vi "test_pattern_recognition.vi"() -> ()   [LabVIEW 2015]
panel:
  out "Matches (pixel) 2":T1(array[cluster])
  in  "Imaginea":path
  in  "Path to template":path
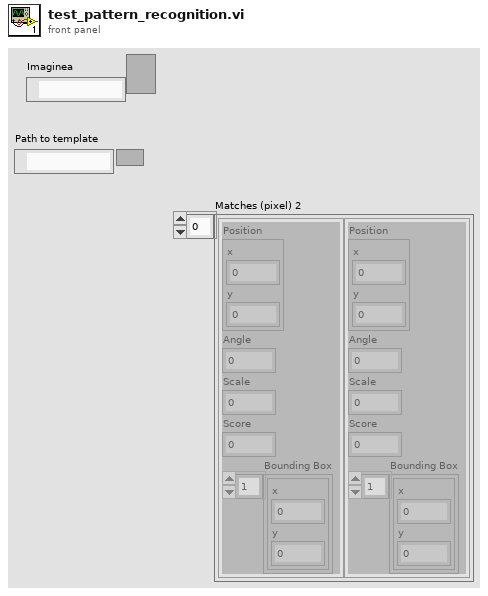
[diagram p1: front panel]
types:
  T1 = cluster{"Position":cluster{"x":sgl, "y":sgl}, "Angle":sgl, "Scale":sgl, "Score":sgl, "Bounding Box":cluster{"x":sgl, "y":sgl}[]}[]
  T2 = typedef "IMAQ Image.ctl" = refnum<image>
  T3 = cluster{"Position":cluster{"x":sgl, "y":sgl}, "Angle":sgl, "Scale":sgl, "Score":sgl, "Bounding Box":cluster{"x":sgl, "y":sgl}[]}
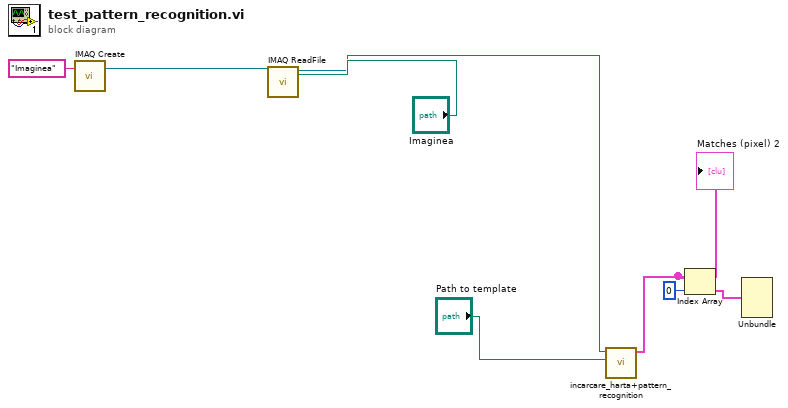
[diagram p0: block diagram]
diagram:
  n1 = call "IMAQ Create"("Image Name"="Imaginea") -> ("New Image"=w5:T2)  [unwired: 4 in, 1 out]
  n2 = call "IMAQ ReadFile"("File Path"="Imaginea", "Image"=w5) -> ("Image Out"=w2:T2)  [unwired: 5 in, 4 out]
  n3 = call "incarcare_harta+pattern_recognition.vi"("Find"="Path to template", "Image 2"=w2) -> ("Matches (pixel)"=w1:T1)  [unwired: 9 in]
  "Matches (pixel) 2" <- w1
  n4 = Index Array(array=w1, index=0) -> (element=w6:T3)
  n5 = Unbundle(w6) -> ()  [unwired: 5 out]
